vi "findFile.vi"(8 "Error In":errorcluster, 9 "Files":refnum<k24>[](array[refnum]), 10 "File Name":string) -> (0 "error out":errorcluster, 2 "File Reference":refnum<k24>)   [LabVIEW 2018, in "GDrive.lvlib"]
doc: "This VI is designed to output a reference to a specific file, given that file's name."
uses:
  GDrive.lvlib
  Y:/UCLA Google Drive/Xavier's Retina MBP/LabVIEW/GDrive/Dependencies/Google.Apis.Drive.v3.dll
  Dependencies/Google.Apis.Drive.v3.dll
panel:
  # "This VI will return a file reference, if the User provides the\nname of the file on the drive. This reference can be mani-\npulated to change various metadata properties of a file."
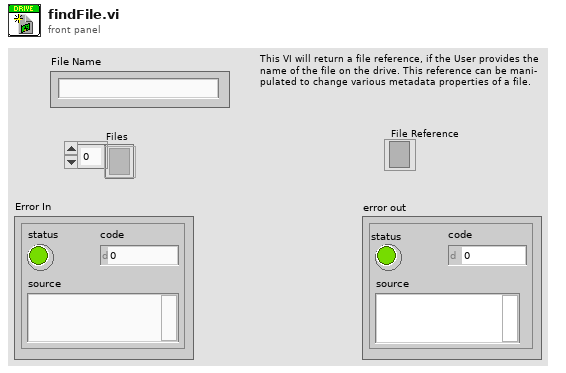
[diagram p1: front panel]
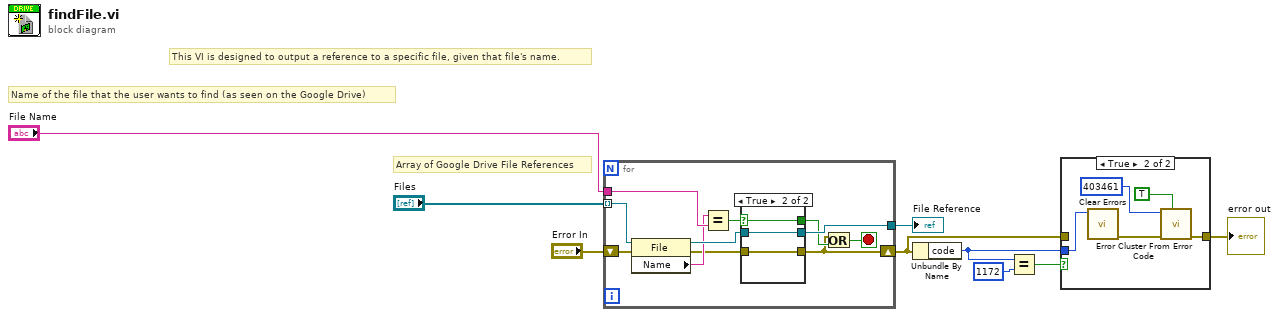
[diagram p0: block diagram]
diagram:
  # "Array of Google Drive File References"
  # "Name of the file that the user wants to find (as seen on the Google Drive)"
  # "This VI is designed to output a reference to a specific file, given that file's name."
  n1 = for {
    tunnel: "Files" -> [w20] mode=indexing
    tunnel: "File Name" -> [w19]
    tunnel: [w18] -> w7
    shift-right: [w11] -> w4
    shift-left: "Error In" -> [w10]
    stop <- w13 stop-if-true
    n2 = property class="File"(reference=w20, error in=w10) -> (reference out=w17:refnum<k24>, error out=w14:errorcluster, "Name"=w15:string)
    n3 = Equal?(x=w15, y=w19) -> (x = y?=w16:bool)
    n4 = case shown="True" w16 {
      selector: w16 -> [w21 w23]
      tunnel: [_ w25] -> w18
      tunnel: w17 -> [_ w25]
      tunnel: [w22 w24] -> w11
      tunnel: w14 -> [w22 w24]
      tunnel: [w21 w23] -> w12
      frame False {
      }
      frame True {
      }
    }
    n5 = Or(x=w11, y=w12) -> (x .or. y?=w13:bool)
  }
  "File Reference" <- w7
  n6 = Unbundle By Name(w4) -> ("code"=w2:i32)
  n7 = Equal?(x=w2, y=1172) -> (x = y?=w5:bool)
  n8 = case shown="True" w5 {
    tunnel: w4 -> [w26 _]
    tunnel: [w26 w31] -> w3
    tunnel: w2 -> [_ w29]
    frame False {
    }
    frame True {
      n9 = call <vilib>:"Clear Errors.vi"("specific error code to clear (0: all)"=w29) -> ("error out"=w30:errorcluster)  [unwired: 5 in, 1 out]
      n10 = call <vilib>:"Error Cluster From Error Code.vi"("show call chain? (False)"=TRUE, "error in (no error)"=w30, "error code (0)"=403461) -> ("error out"=w31:errorcluster)  [unwired: 6 in]
    }
  }
  "error out" <- w3
